vi "Serial Client.vi"() -> ()   [LabVIEW 2017]
uses:
  <vilib>/Instr/_visa.llb/VISA Configure Serial Port (Instr).vi
panel:
  out "错误输出":errorcluster
  in  "布尔":bool
  out "读取缓冲区":string
  out "VISA资源名称输出":refnum<visa-resource-name>
  in  "VISA资源名称 2":refnum<visa-resource-name>
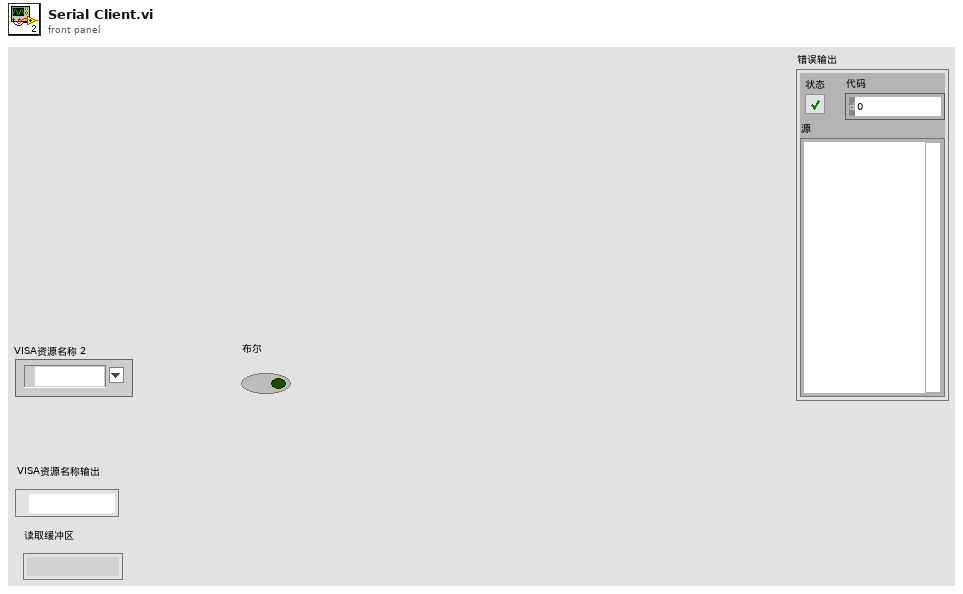
[diagram p1: front panel]
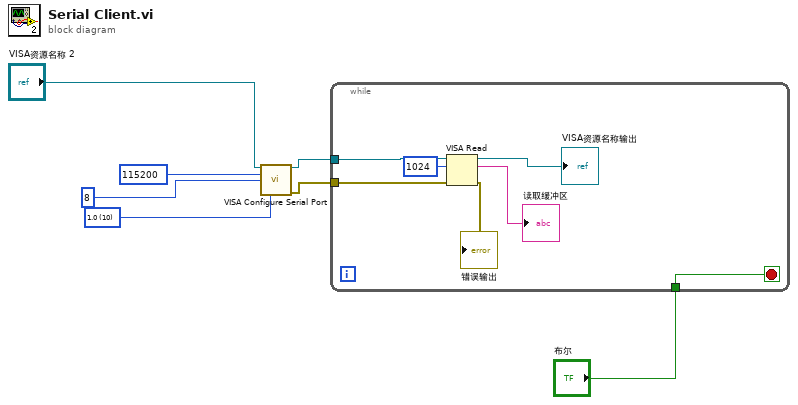
[diagram p0: block diagram]
diagram:
  w4 = u16 10 items=["1.0"=10, "1.5"=15, "2.0"=20] ("stop bits (10: 1 bit)")
  n1 = call-poly "VISA Configure Serial Port"("VISA resource name"="VISA资源名称 2", "baud rate (9600)"=u32 115200, "data bits (8)"=u16 8, "stop bits (10: 1 bit)"=w4) -> ("VISA resource name out"=w3:refnum<visa-resource-name>, "error out"=w1:errorcluster)  [unwired: 10 in]
  n2 = while {
    tunnel: w3 -> [w14]
    tunnel: "布尔" -> [w11]
    tunnel: w1 -> [w9]
    stop <- w11 stop-if-true
    n3 = VISA Read(VISA resource name=w14, byte count=u32 1024 ("字节总数"), error in (no error)=w9) -> (VISA resource name out=→"VISA资源名称输出":refnum<visa-resource-name>, read buffer=→"读取缓冲区":string, error out=→"错误输出":errorcluster)  [unwired: 1 out]
  }
